vi "Temp To F.vi"() -> ()   [LabVIEW 2020]
panel:
  out "F":dbl
  in  "T":i8
  # "Conversion Temp to F"
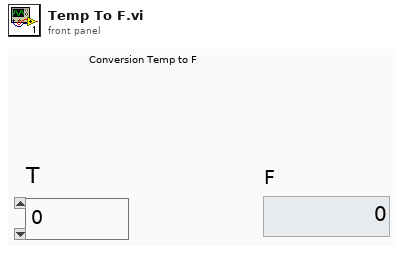
[diagram p1: front panel]
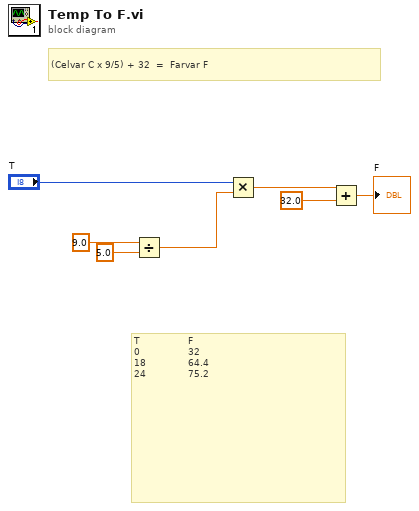
[diagram p0: block diagram]
diagram:
  # "T                F\n0                32\n18              64.4\n24              75.2"
  # "(Celvar C x 9/5) + 32  =  Farvar F"
  n1 = Divide(x=9.0, y=5.0) -> (x/y=w4:dbl)
  n2 = Multiply(x="T", y=w4) -> (x*y=w3:dbl)
  n3 = Add(x=w3, y=32.0) -> (x+y=→"F":dbl)
